vi "General Client.vi"() -> ()   [LabVIEW 2018]
uses:
  <vilib>/LabVIEW Open Source Project/MQTT Client/Client class/Client.lvclass/Client.ctl
  <vilib>/LabVIEW Open Source Project/MQTT Connection/MQTT_Base/Base Class/MQTT_Base.lvclass/MQTT_Base.ctl
  <vilib>/LabVIEW Open Source Project/Connection/Connection.TCP/Connection.TCP.lvclass
  C:/Program Files (x86)/National Instruments/LabVIEW 2018/vi.lib/LabVIEW Open Source Project/Connection/Connection/Connection.lvclass
  <vilib>/LabVIEW Open Source Project/MQTT Client/Client class/Client.lvclass
  C:/Program Files (x86)/National Instruments/LabVIEW 2018/vi.lib/LabVIEW Open Source Project/MQTT Connection/MQTT_Base/Base Class/MQTT_Base.lvclass
  <vilib>/LabVIEW Open Source Project/MQTT Control Packets/Control Packets/PUBLISH/PUBLISH.lvclass
  <vilib>/LabVIEW Open Source Project/MQTT Connection/MQTT_Base/Base Class/MQTT_Base.lvclass
  <vilib>/LabVIEW Open Source Project/Connection/Connection.LocalQueue/Connection.LocalQueue.lvclass
  <vilib>/LabVIEW Open Source Project/Connection/Connection/Connection.lvclass
panel:
  in  "Stop Client":bool
  out "last error":errorcluster
  in  "Tab Control":enum32{"MQTT", "TCP/IP"}(tab)
  in  "Connection":bool
  in  "broker address":string(combo)="test.mosquitto.org"
  in  "Command\nTopic Name":string="SPARC4 COMMAND"
  in  "Client Command":string
  out "Published":bool
  out "Status Payload":u8[](array[numeric]) format="%08b"
  out "Received \nStatus":string
  in  "Status\nTopic Name":string="SPARC4 STATUS"
  in  "Status Subscribe":bool
  out "Unsuback":bool
  out "Suback":bool
  in  "clear status":bool
  # "CLIENT COMMAND"
  # "CLIENT RECEIVED STATUS"
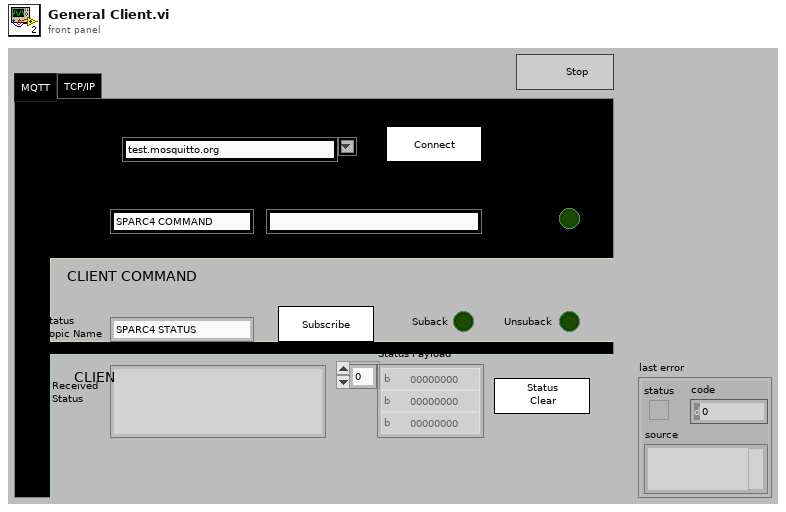
[diagram p1: front panel]
types:
  T1 = typedef "MQTT Client.lvlib/Client.lvclass/Public Events -- cluster.ctl" = cluster{"Connection Status":refnum<user-event>, "Connected":refnum<user-event>, "Application Message":refnum<user-event>}
  T2 = typedef "MQTT Base.lvlib/MQTT_Base.lvclass/Public Events -- cluster.ctl" = cluster{"Stop Event":refnum<user-event>, "Error Event":refnum<user-event>, "Inbound Message":refnum<user-event>}
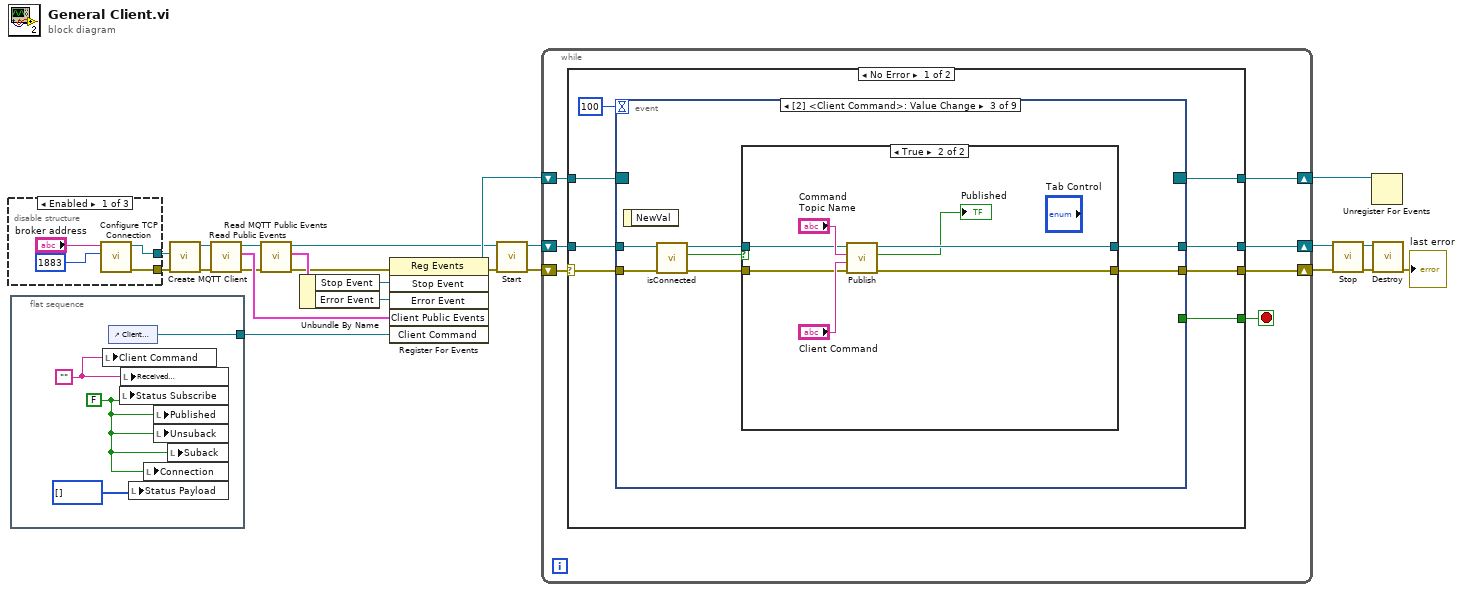
[diagram p0: block diagram]
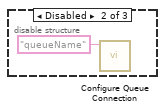
[diagram p2: hidden frame]
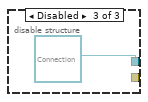
[diagram p3: hidden frame]
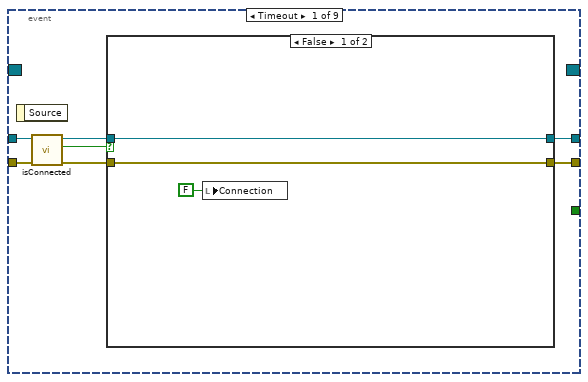
[diagram p4: hidden frame]
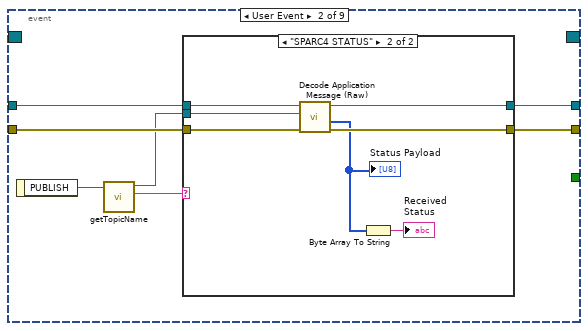
[diagram p6: hidden frame]
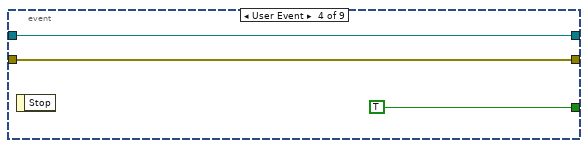
[diagram p9: hidden frame]
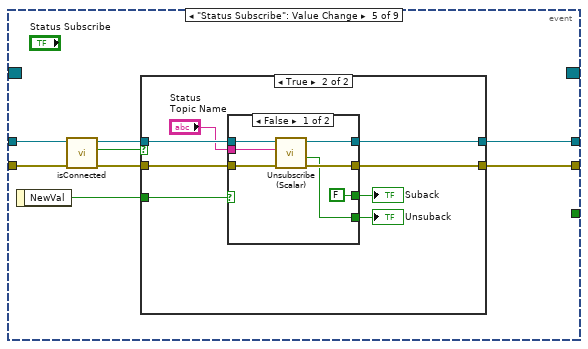
[diagram p10: hidden frame]
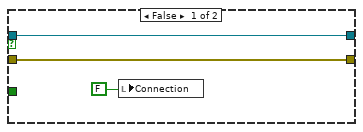
[diagram p11: hidden frame]
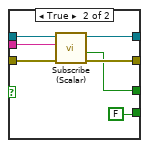
[diagram p12: hidden frame]
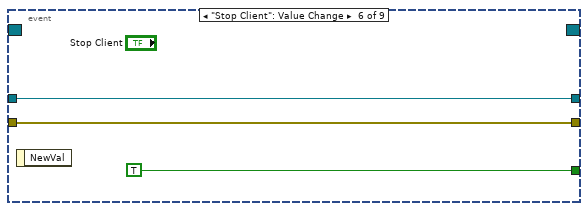
[diagram p13: hidden frame]
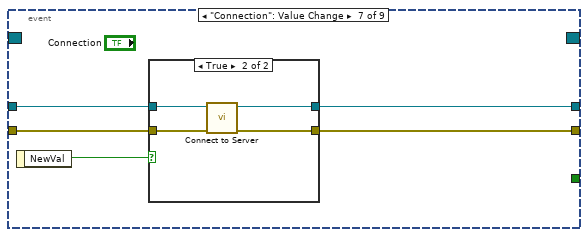
[diagram p14: hidden frame]
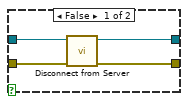
[diagram p15: hidden frame]
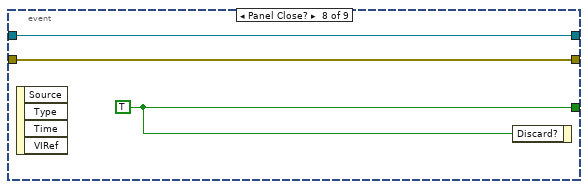
[diagram p16: hidden frame]
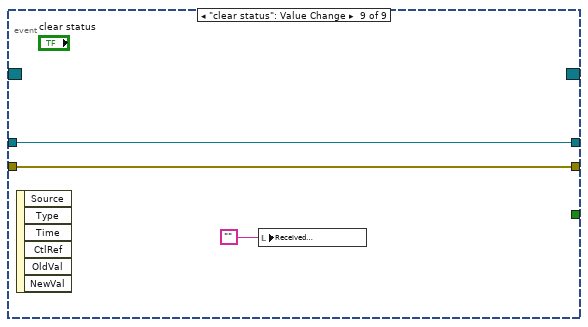
[diagram p17: hidden frame]
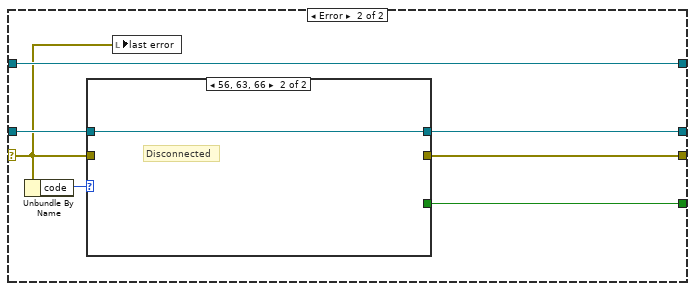
[diagram p18: hidden frame]
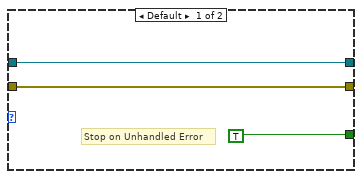
[diagram p19: hidden frame]
diagram:
  n1 = disable-structure shown="Enabled" {
    disable-tunnel: [w26 _ refnum<class "Connection.lvclass"> refnum ("Connection Configuration")] -> w23
    disable-tunnel: [w24 _ _] -> w1
    frame Enabled {
      n2 = call <vilib>:"Configure TCP Connection.vi"("remote port (80)"=u16 1883, "address (localhost)"="broker address") -> ("error out"=w24:errorcluster, "Connection.TCP"=w26:refnum<class "Connection.TCP.lvclass">)  [unwired: 8 in]
    }
    frame Disabled {
      n3 = call <vilib>:"Configure Queue Connection.vi"("Queue Name"="queueName") -> ()  [unwired: 9 in, 2 out]
    }
    frame Disabled {
    }
  }
  n4 = flat-sequence {
    tunnel: [w33] -> w2
    frame #0 {
      w30 = FALSE
      w32 = ""
      n5 = local write "Client Command"(w32) -> ()
      n6 = control-ref of="Client Command"() -> (w33:refnum<vi>)
      n7 = local write "Status Subscribe"(w30) -> ()
      n8 = local write "Received \nStatus"(w32) -> ()
      n9 = local write "Status Payload"(u8[] [] ("Status Payload")) -> ()
      n10 = local write "Connection"(w30) -> ()
      n11 = local write "Published"(w30) -> ()
      n12 = local write "Unsuback"(w30) -> ()
      n13 = local write "Suback"(w30) -> ()
    }
  }
  n14 = call <vilib>:"Create MQTT Client.vi"("error in (no error)"=w1, "Connection Configuration"=w23) -> ("error out"=w5:errorcluster, "Client out"=w3:refnum<class "Client.lvclass">)  [unwired: 8 in]
  n15 = call <vilib>:"Read Public Events.vi"("error in (no error)"=w5, "Client in"=w3) -> ("error out"=w6:errorcluster, "Client Public Events"=w8:T1, "Client out"=w4:refnum<class "Client.lvclass">)  [unwired: 7 in]
  n16 = call <vilib>:"Read MQTT Public Events.vi"("error in (no error)"=w6, "MQTT_Base in"=w4) -> ("error out"=w7:errorcluster, "MQTT Public Events"=w15:T2, "MQTT_Base out"=w10:refnum<class "Client.lvclass">)  [unwired: 7 in]
  n17 = Unbundle By Name(w15) -> ("Stop Event"=w13:refnum<user-event>, "Error Event"=w14:refnum<user-event>)
  n18 = register-events(error in=w7, w13, w14, w8, w2) -> (reference out=w11:refnum<event-registration>, error out=w9:errorcluster)  [unwired: 1 in]
  n19 = call <vilib>:"Start.vi"("error in (no error)"=w9, "MQTT_Base in"=w10) -> ("error out"=w21:errorcluster, "MQTT_Base out"=w20:refnum<class "Client.lvclass">)  [unwired: 7 in, 1 out]
  n20 = while {
    shift-right: [w39] -> w12
    shift-left: w11 -> [w40]
    shift-right: [w36] -> w17
    shift-left: w20 -> [w37]
    shift-right: [w38] -> w19
    shift-left: w21 -> [w34]
    stop <- w35 stop-if-true
    n21 = case shown="No Error" w34 {
      selector: w34 -> [w41 w151]
      tunnel: w40 -> [w48 w157]
      tunnel: [w47 w157] -> w39
      tunnel: [w46 w153] -> w38
      tunnel: w37 -> [w44 w155]
      tunnel: [w43 w154] -> w36
      tunnel: [w42 w152] -> w35
      frame No Error {
        n22 = event shown="[2] <Client Command>: Value Change" {
          selector: w48 -> [_ _ _ _ _ _ _ _ _]
          dyn-events: [_ _ _ _ _ _ _ _ _] -> w47
          timeout: 100 -> [_ _ _ _ _ _ _ _ _]
          tunnel: w41 -> [w51 w64 w82 w95 w102 w130 w132 w145 w149]
          tunnel: [w54 w62 w78 w95 w97 w130 w133 w145 w149] -> w46
          tunnel: [_ _ _ TRUE _ TRUE _ w147 _] -> w42
          tunnel: w44 -> [w53 w65 w83 w93 w103 w131 w136 w146 w150]
          tunnel: [w55 w61 w77 w93 w96 w131 w134 w146 w150] -> w43
          event Timeout {
            n23 = event-data() -> ()  [unwired: 1 in, 1 out]
            n24 = call <vilib>:"isConnected.vi"("error in (no error)"=w51, "Client in"=w53) -> ("error out"=w50:errorcluster, "connected"=w49:bool, "Client out"=w52:refnum<class "Client.lvclass">)  [unwired: 7 in]
            n25 = case shown="False" w49 {
              tunnel: [w58 w60] -> w55
              tunnel: [w57 w59] -> w54
              tunnel: w52 -> [w58 w60]
              tunnel: w50 -> [w57 w59]
              frame False {
                n26 = local write "Connection"(FALSE ("Connection")) -> ()
              }
              frame True {
              }
            }
          }
          event User Event {
            n27 = event-data() -> ("PUBLISH"=w67:refnum<class "PUBLISH.lvclass">)  [unwired: 1 in]
            n28 = call <vilib>:"getTopicName.vi"("PUBLISH in"=w67) -> ("Topic"=w66:string, "PUBLISH out"=w63:refnum<class "PUBLISH.lvclass">)  [unwired: 8 in, 1 out]
            n29 = case shown="\"SPARC4 STATUS\"" w66 {
              tunnel: w65 -> [w69 w76]
              tunnel: w64 -> [w68 w75]
              tunnel: w63 -> [_ w74]
              tunnel: [w68 w73] -> w62
              tunnel: [w69 w72] -> w61
              frame Default {
              }
              frame "SPARC4 STATUS" {
                n30 = call <vilib>:"Decode Application Message (Raw).vi"("error in (no error)"=w75, "PUBLISH"=w74, "Client in"=w76) -> ("error out"=w73:errorcluster, "Payload"=w70:u8[], "Client out"=w72:refnum<class "Client.lvclass">)  [unwired: 5 in, 1 out]
                "Status Payload" <- w70
                n31 = Byte Array To String(unsigned byte array=w70) -> (string=→"Received \nStatus":string)
              }
            }
          }
          event Value Change {
            n32 = event-data() -> ()  [unwired: 1 in, 1 out]
            n33 = call <vilib>:"isConnected.vi"("error in (no error)"=w82, "Client in"=w83) -> ("error out"=w79:errorcluster, "connected"=w81:bool, "Client out"=w80:refnum<class "Client.lvclass">)  [unwired: 7 in]
            n34 = case shown="True" w81 {
              tunnel: w80 -> [w84 w89]
              tunnel: w79 -> [w85 w90]
              tunnel: [w85 w88] -> w78
              tunnel: [w84 w87] -> w77
              frame False {
              }
              frame True {
                n35 = call <vilib>:"Publish.vi"("error in (no error)"=w90, "Payload"="Client Command", "Topic Name (empty: Payload name)"="Command\nTopic Name", "Client in"=w89) -> ("error out"=w88:errorcluster, "Published"=→"Published":bool, "Client out"=w87:refnum<class "Client.lvclass">)  [unwired: 5 in]
              }
            }
          }
          event User Event {
            n36 = event-data() -> ()  [unwired: 1 in, 1 out]
          }
          event "Status Subscribe": Value Change {
            n37 = event-data() -> ("NewVal"=w98:bool)  [unwired: 1 in]
            n38 = call <vilib>:"isConnected.vi"("error in (no error)"=w102, "Client in"=w103) -> ("error out"=w99:errorcluster, "connected"=w101:bool, "Client out"=w100:refnum<class "Client.lvclass">)  [unwired: 7 in]
            n39 = case shown="True" w101 {
              tunnel: w100 -> [w106 w114]
              tunnel: w99 -> [w105 w113]
              tunnel: w98 -> [_ w112]
              tunnel: [w105 w110] -> w97
              tunnel: [w106 w109] -> w96
              frame False {
                n40 = local write "Connection"(FALSE) -> ()
              }
              frame True {
                n41 = case shown="False" w112 {
                  tunnel: w114 -> [w120 w128]
                  tunnel: w113 -> [w121 w127]
                  tunnel: "Status\nTopic Name" -> [w115 w126]
                  tunnel: [w118 w125] -> w110
                  tunnel: [w119 w124] -> w109
                  tunnel: [FALSE w123] -> w108
                  tunnel: [w117 FALSE] -> w107
                  frame False {
                    n42 = call <vilib>:"Unsubscribe (Scalar).vi"("error in (no error)"=w121, "Topic Filter"=w115, "Client in"=w120) -> ("error out"=w118:errorcluster, "Ack"=w117:bool, "Client out"=w119:refnum<class "Client.lvclass">)  [unwired: 6 in]
                  }
                  frame True {
                    n43 = call <vilib>:"Subscribe (Scalar).vi"("error in (no error)"=w127, "Topic Filter"=w126, "Client in"=w128) -> ("error out"=w125:errorcluster, "Ack"=w123:bool, "Client out"=w124:refnum<class "Client.lvclass">)  [unwired: 6 in]
                  }
                }
                "Unsuback" <- w107
                "Suback" <- w108
              }
            }
          }
          event "Stop Client": Value Change {
            n44 = event-data() -> ()  [unwired: 1 in, 1 out]
          }
          event "Connection": Value Change {
            n45 = event-data() -> ("NewVal"=w135:bool)  [unwired: 1 in]
            n46 = case shown="True" w135 {
              tunnel: w136 -> [w140 w144]
              tunnel: [w139 w141] -> w134
              tunnel: [w138 w142] -> w133
              tunnel: w132 -> [w137 w143]
              frame False {
                n47 = call <vilib>:"Disconnect from Server.vi"("error in (no error)"=w137, "Client in"=w140) -> ("error out"=w138:errorcluster, "Client out"=w139:refnum<class "Client.lvclass">)  [unwired: 7 in, 1 out]
              }
              frame True {
                n48 = call <vilib>:"Connect to Server.vi"("error in (no error)"=w143, "Client in"=w144) -> ("error out"=w142:errorcluster, "Client out"=w141:refnum<class "Client.lvclass">)  [unwired: 6 in, 2 out]
              }
            }
          }
          event Panel Close? {
            w147 = TRUE
            n49 = event-data() -> ()  [unwired: 1 in, 4 out]
            n50 = event-data("Discard?"=w147) -> ()  [unwired: 1 in, 1 out]
          }
          event "clear status": Value Change {
            n51 = event-data() -> ()  [unwired: 1 in, 6 out]
            n52 = local write "Received \nStatus"("") -> ()
          }
        }
      }
      frame Error {
        n53 = Unbundle By Name(w151) -> ("code"=w156:i32)
        n54 = case shown="56, 63, 66" w156 {
          tunnel: w155 -> [w160 w161]
          tunnel: [w160 w161] -> w154
          tunnel: w151 -> [w159 _]
          tunnel: [w159 _] -> w153
          tunnel: [TRUE _] -> w152
          frame Default {
            # "Stop on Unhandled Error"
          }
          frame 56, 63, 66 {
            # "Disconnected"
          }
        }
        n55 = local write "last error"(w151) -> ()
      }
    }
  }
  n56 = call <vilib>:"Stop.vi"("error in (no error)"=w19, "MQTT_Base in"=w17) -> ("error out"=w18:errorcluster, "MQTT_Base out"=w16:refnum<class "Client.lvclass">)  [unwired: 7 in, 1 out]
  n57 = Unregister For Events(event registration refnum=w12) -> ()  [unwired: 1 in, 1 out]
  n58 = call <vilib>:"Destroy.vi"("error in (no error)"=w18, "MQTT_Base in"=w16) -> ("error out"=→"last error":errorcluster)  [unwired: 8 in, 1 out]
